vi "Contour Line_Find Intersected Edges (row).vi"(7 "row":i32, 8 "height":dbl, 9 "Z":dbl[][](array[numeric]), 10 "Y":dbl[][](array[numeric]), 11 "X":dbl[][](array[numeric])) -> (2 "Intersected Edges":T1(array[cluster]), 3 "Contour Points":cluster{"x":dbl, "y":dbl}[](array[cluster]))   [LabVIEW 2020, in "NI_AAL_Geometry.lvlib"]
uses:
  <vilib>/Analysis/NI_AAL_Geometry.lvlib
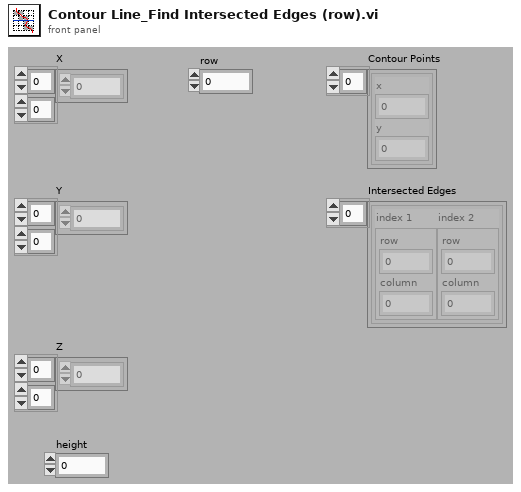
[diagram p1: front panel]
types:
  T1 = cluster{"index 1":cluster{"row":i32, "column":i32}, "index 2":cluster{"row":i32, "column":i32}}[]
  T2 = cluster{"index 1":cluster{"row":i32, "column":i32}, "index 2":cluster{"row":i32, "column":i32}}
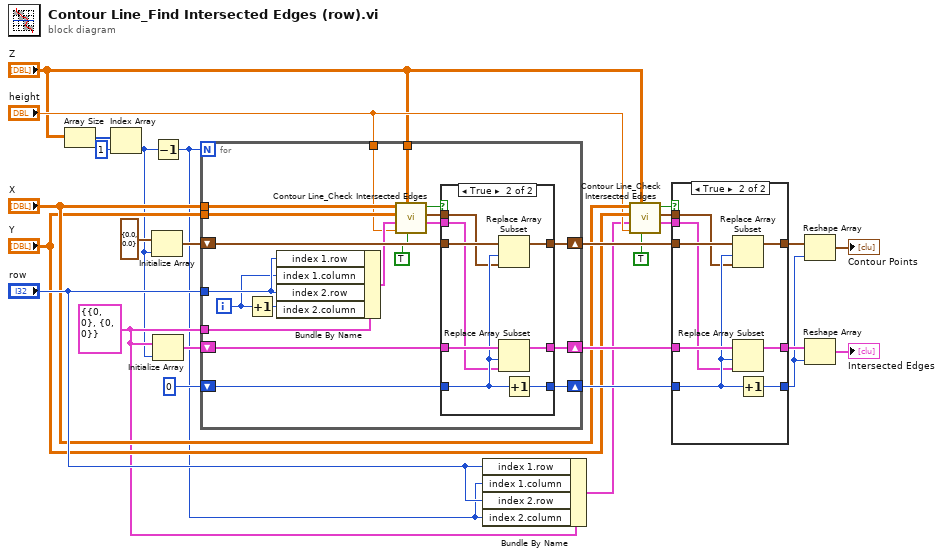
[diagram p0: block diagram]
diagram:
  w7 = T2 {"index 1"={"row"=0, "column"=0}, "index 2"={"row"=0, "column"=0}} ("intersected edge")
  n1 = Array Size(array="Z") -> (size(s)=w27:i32[])
  n2 = Index Array(array=w27, index=1) -> (element=w4:i32)
  n3 = Initialize Array(cluster{"x":dbl, "y":dbl} {"x"=0.0, "y"=0.0} ("contour point"), w4) -> (w24:cluster{"x":dbl, "y":dbl}[])
  n4 = Decrement(x=w4) -> (x-1=w3:i32)
  n5 = Initialize Array(w7, w4) -> (w23:T1)
  n6 = for {
    N: w3 -> [_]
    tunnel: "row" -> [w37]
    tunnel: "height" -> [w31]
    tunnel: "X" -> [w39]
    tunnel: "Y" -> [w38]
    shift-right: [w45] -> w21
    shift-left: w24 -> [w46]
    shift-right: [w43] -> w20
    shift-left: w23 -> [w44]
    shift-right: [w40] -> w19
    shift-left: 0 -> [w42]
    tunnel: w7 -> [w41]
    tunnel: "Z" -> [w28]
    i -> [w35]
    n7 = Increment(x=w35) -> (x+1=w36:i32)
    n8 = Bundle By Name(cluster=w41, "index 1.row"=w37, "index 1.column"=w35, "index 2.row"=w37, "index 2.column"=w36) -> (w33:T2)
    n9 = call <vilib>:"Contour Line_Check Intersected Edges.vi"("row? (F)"=TRUE, "Z"=w28, "height"=w31, "edge in"=w33, "Y"=w38, "X"=w39) -> ("edge out"=w32:T2, "contour point"=w34:cluster{"x":dbl, "y":dbl}, "intersected?"=w30:bool)  [unwired: 3 out]
    n10 = case shown="True" w30 {
      tunnel: w46 -> [w49 w57]
      tunnel: [w49 w56] -> w45
      tunnel: w44 -> [w48 w55]
      tunnel: [w48 w54] -> w43
      tunnel: w42 -> [w47 w53]
      tunnel: [w47 w52] -> w40
      tunnel: w34 -> [_ w51]
      tunnel: w32 -> [_ w50]
      frame False {
      }
      frame True {
        n11 = Replace Array Subset(array=w57, new element=w51, index=w53) -> (w56:cluster{"x":dbl, "y":dbl}[])
        n12 = Replace Array Subset(array=w55, new element=w50, index=w53) -> (w54:T1)
        n13 = Increment(x=w53) -> (x+1=w52:i32)
      }
    }
  }
  n14 = Bundle By Name(cluster=w7, "index 1.row"="row", "index 1.column"=w3, "index 2.row"="row", "index 2.column"=w3) -> (w6:T2)
  n15 = call <vilib>:"Contour Line_Check Intersected Edges.vi"("row? (F)"=TRUE, "Z"="Z", "height"="height", "edge in"=w6, "Y"="Y", "X"="X") -> ("edge out"=w8:T2, "contour point"=w9:cluster{"x":dbl, "y":dbl}, "intersected?"=w5:bool)  [unwired: 3 out]
  n16 = case shown="True" w5 {
    tunnel: w21 -> [w59 w68]
    tunnel: w20 -> [w60 w67]
    tunnel: w19 -> [w58 w66]
    tunnel: [w58 w61] -> w16
    tunnel: [w60 w65] -> w17
    tunnel: [w59 w64] -> w18
    tunnel: w9 -> [_ w63]
    tunnel: w8 -> [_ w62]
    frame False {
    }
    frame True {
      n17 = Replace Array Subset(array=w68, new element=w63, index=w66) -> (w64:cluster{"x":dbl, "y":dbl}[])
      n18 = Replace Array Subset(array=w67, new element=w62, index=w66) -> (w65:T1)
      n19 = Increment(x=w66) -> (x+1=w61:i32)
    }
  }
  n20 = Reshape Array(w18, w16) -> (→"Contour Points":cluster{"x":dbl, "y":dbl}[])
  n21 = Reshape Array(w17, w16) -> (→"Intersected Edges":T1)
